vi "Write Instrument finder Done boolean to Ref.vi"(8 "error in (no error)":errorcluster, 10 "done":bool, 11 "Controller in":refnum<class "Controller.lvclass">) -> (0 "error out":errorcluster, 3 "Controller out":refnum<class "Controller.lvclass">)   [LabVIEW 2014, in "Controller.lvclass"]
uses:
  Controller.lvclass
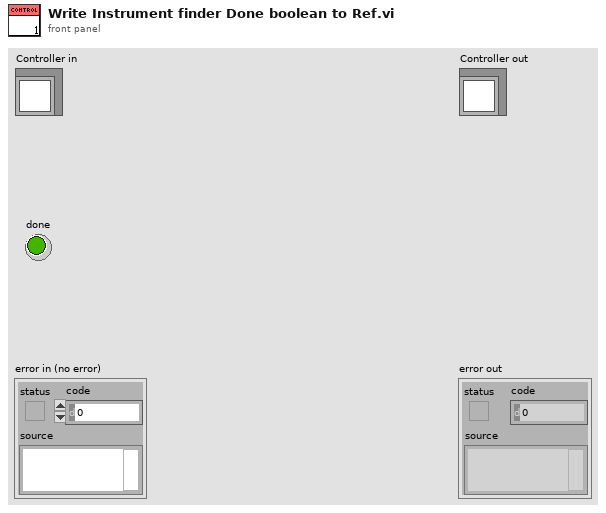
[diagram p1: front panel]
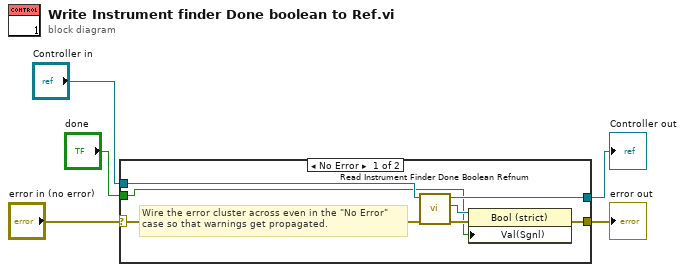
[diagram p0: block diagram]
diagram:
  n1 = case shown="No Error" "error in (no error)" {
    selector: "error in (no error)" -> [w10 w14]
    tunnel: [w7 w14] -> w4
    tunnel: [w11 w13] -> w2
    tunnel: "Controller in" -> [w12 w13]
    tunnel: "done" -> [w6 _]
    frame No Error {
      # "Wire the error cluster across even in the \"No Error\"\ncase so that warnings get propagated."
      n2 = call-dynamic "Read Instrument Finder Done Boolean Refnum.vi"("error in (no error)"=w10, "Controller in"=w12) -> ("error out"=w8:errorcluster, "Instrument Finder Done Boolean Refnum"=w9:refnum<vi>, "Controller out"=w11:refnum<class "Controller.lvclass">)  [unwired: 7 in]
      n3 = property class="Bool (strict)"(reference=w9, error in=w8, "Val(Sgnl)"=w6) -> (error out=w7:errorcluster)  [unwired: 1 out]
    }
    frame Error {
    }
  }
  "error out" <- w4
  "Controller out" <- w2
